vi "Set Reley.vi"(8 "Reverse":bool, 9 "Forward":bool, 11 "refnum name":string="My Relay RefNum") -> ()   [LabVIEW 2014]
doc: "Sets a reley in three states forwards, reverse and off."
uses:
  <vilib>/Rock Robotics/WPI/Relay/WPI_RelayValue.ctl
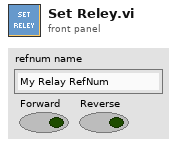
[diagram p1: front panel]
types:
  T1 = typedef "WPI_RelayValue.ctl" = enum16{"Off", "On", "Forward", "Reverse"}
  T2 = typedef "WPI_RelayDevRef.ctl" = cluster{"DevStatus":errorcluster, "Relay Channel":T3, "Digital Module":T4, "Relay Direction":T5}
  T3 = typedef "FPGA_DIORelayChannel.ctl" = enum8{"Relay 1", "Relay 2", "Relay 3", "Relay 4", "Relay 5", "Relay 6", "Relay 7", "Relay 8", "Invalid"}
  T4 = typedef "FPGA_TypedefDigitalModule.ctl" = enum16{"Digital Module 1", "Digital Module 2"}
  T5 = typedef "WPI_RelayDirection.ctl" = enum16{"Both directions", "Forward only", "Reverse only"}
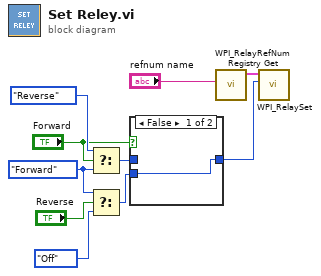
[diagram p0: block diagram]
diagram:
  w6 = WPI_RelayValue."Forward" ("RelayValue")
  n1 = Select(t=WPI_RelayValue."Reverse" ("RelayValue"), s="Forward", f=w6) -> (s? t:f=w10:T1)
  n2 = Select(t=w6, s="Reverse", f=WPI_RelayValue."Off" ("RelayValue")) -> (s? t:f=w9:T1)
  n3 = case shown="False" "Forward" {
    tunnel: [w11 w12] -> w4
    tunnel: w10 -> [_ w12]
    tunnel: w9 -> [w11 _]
    frame False {
    }
    frame True {
    }
  }
  n4 = call <vilib>:"WPI_RelayRefNum Registry Get.vi"("refnum name"="refnum name") -> ("RelayDevRef"=w5:T2)  [unwired: 9 in, 1 out]
  n5 = call <vilib>:"WPI_RelaySet.vi"("RelayValue"=w4, "RelayDevRef"=w5) -> ()  [unwired: 8 in, 2 out]
